vi "test.vi"() -> ()   [LabVIEW 2023]
panel:
  in  "String 2":string
  in  "String":string
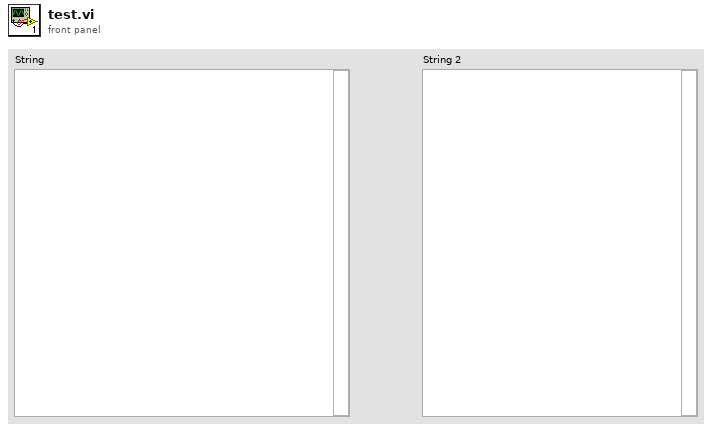
[diagram p1: front panel]
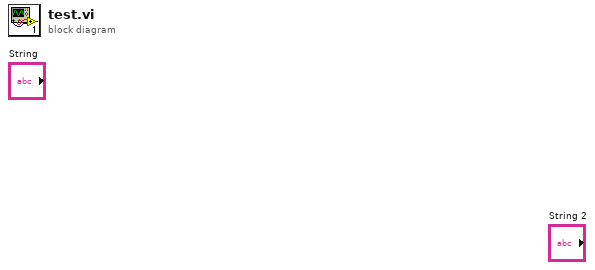
[diagram p0: block diagram]
diagram:
